vi "GetAllControlRefs_Ref.vi"(4 "Add Array Ctls? [T]":bool=TRUE, 6 "Add Cluster Ctls? [T]":bool=TRUE, 8 "error in (no error)":errorcluster, 11 "VI Ref":refnum<vi>) -> (0 "error out":errorcluster, 3 "CtlLookup Out":T1)   [LabVIEW 2020, in "CtlReferences.lvlib" / "CtlReferences.lvclass"]
doc: "generate all of the Control Refs for a give VI"
uses:
  CtlReferences.lvclass
  TypeDefs/CtlLookup.ctl
  CtlReferences.lvclass/CtlReferences.ctl
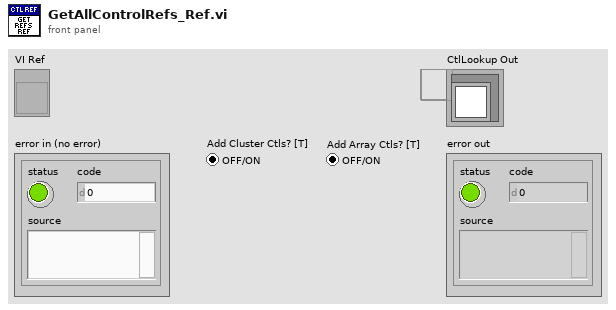
[diagram p1: front panel]
types:
  T1 = typedef "CtlReferences.lvlib/CtlReferences.lvclass/CtlLookup.ctl" = refnum<data-value>
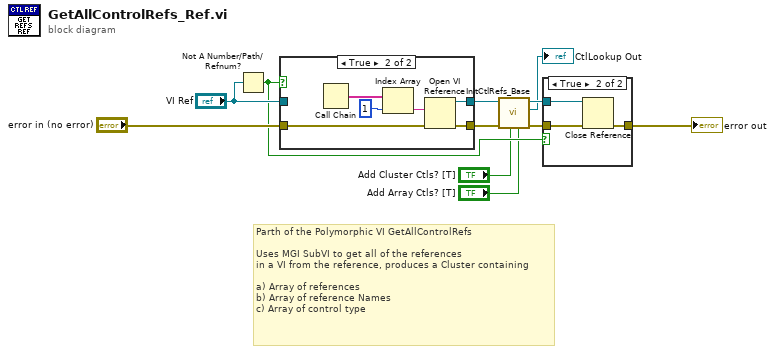
[diagram p0: block diagram]
diagram:
  # "Parth of the Polymorphic VI GetAllControlRefs\n\nUses MGI SubVI to get all of the references \nin a VI from the reference, produces a Cluster containing\n\na) Array of references\nb) Array of reference Names\nc) Array of control type"
  n1 = Not A Number/Path/Refnum?(number/path/refnum="VI Ref") -> (NaN/Path/Refnum?=w3:bool)
  n2 = case shown="True" w3 {
    tunnel: "error in (no error)" -> [w13 w16]
    tunnel: [w13 w15] -> w8
    tunnel: "VI Ref" -> [w12 _]
    tunnel: [w12 w14] -> w7
    frame False {
    }
    frame True {
      n3 = Call Chain() -> (call chain=w18:string[])
      n4 = Index Array(array=w18, index=1) -> (element=w17:string)
      n5 = Open VI Reference(vi path=w17, error in (no error)=w16) -> (vi reference=w14:refnum<vi>, error out=w15:errorcluster)  [unwired: 4 in]
    }
  }
  n6 = call "InitCtlRefs_Base.vi"("Add Array Ctls?"="Add Array Ctls? [T]", "Add Cluster Ctls?"="Add Cluster Ctls? [T]", "error in (no error)"=w8, "VI in"=w7) -> ("error out"=w6:errorcluster, "Data Value Reference out"=→"CtlLookup Out":T1, "VI out"=w5:refnum<vi>)  [unwired: 5 in]
  n7 = case shown="True" w3 {
    tunnel: w6 -> [w20 w23]
    tunnel: [w20 w22] -> w11
    tunnel: w5 -> [_ w21]
    frame False {
    }
    frame True {
      n8 = Close Reference(reference=w21, error in (no error)=w23) -> (error out=w22:errorcluster)
    }
  }
  "error out" <- w11
